vi "ELI-TriScope-StageController-V1.0.0.vi"() -> ()   [LabVIEW 2011]
uses:
  D:/Program Files/New Focus/New Focus Picomotor Application/Samples/CmdLib.dll
panel:
  in  "CurrentAngleA":dbl caption="CurrentAngle:" format="%.3g"
  in  "步长（nm）":dbl=31.75 format="%.2f"
  in  "relative position":i32=100
  in  "position profile":T1={"profileVelocity"=1000, "profileAcceleration"=10000, "profileDeceleration"=10000}
  in  "homeA":bool
  in  "ZeroA":bool
  in  "GoA":bool
  in  "AngleA":dbl=-18.0 caption="Angle:" format="%.3g"
  in  "file (use dialog)":path=path "C:/Users/Administrator/Desktop/stage2.txt"
  out "Current PositionY":dbl caption="Position:" format="%.3g"
  in  "JogY+":bool
  in  "JogY-":bool
  in  "StopY":bool
  in  "GoY":bool
  in  "Relative MoveY":dbl=3.0 caption="Step:" format="%.3g"
  out "Current PositionX":dbl caption="Position:" format="%.3g"
  in  "JogX+":bool
  in  "JogX-":bool
  in  "StopX":bool
  in  "GoX":bool
  in  "Relative MoveX":dbl=3.0 caption="Step:" format="%.3g"
  out "XYZ motors connect":bool
  in  "GoX 2":bool
  in  "GoY 2":bool
  in  "homeX":bool
  in  "ZeroX":bool
  in  "homeY":bool
  in  "ZeroY":bool
  out "Position:":dbl format="%.3g"
  in  "JogZ+":bool
  in  "JogZ-":bool
  in  "StopZ":bool
  in  "GoZ":bool
  in  "Relative MoveZ":dbl=3.0 caption="Step:" format="%.3g"
  in  "GoZ 2":bool
  in  "homeZ":bool
  in  "ZeroZ":bool
  out "targetPosZ":i32=88
  out "targetPosY":i32=13
  out "targetPosX":i32=-3455
  out "offsetZ":i32=-88
  out "offsetY":i32=-13
  out "offsetX":i32=3455
  out "CC Min":u32
  out "Exp. out":i32
  out "Clearing modes":i32=3
  out "Full CCD Height":i32=1200
  out "Full CCD Width":i32=1200
  out "Y Binning":u32=1
  out "X Binning":u32=1
  # "X motor"
  # "（um）"
  # "（um）"
  # "Y motor"
  # "（um）"
  # "（um）"
  # "Z motor"
  # "（um）"
  # "（um）"
  # "A motor"
  # "（°）"
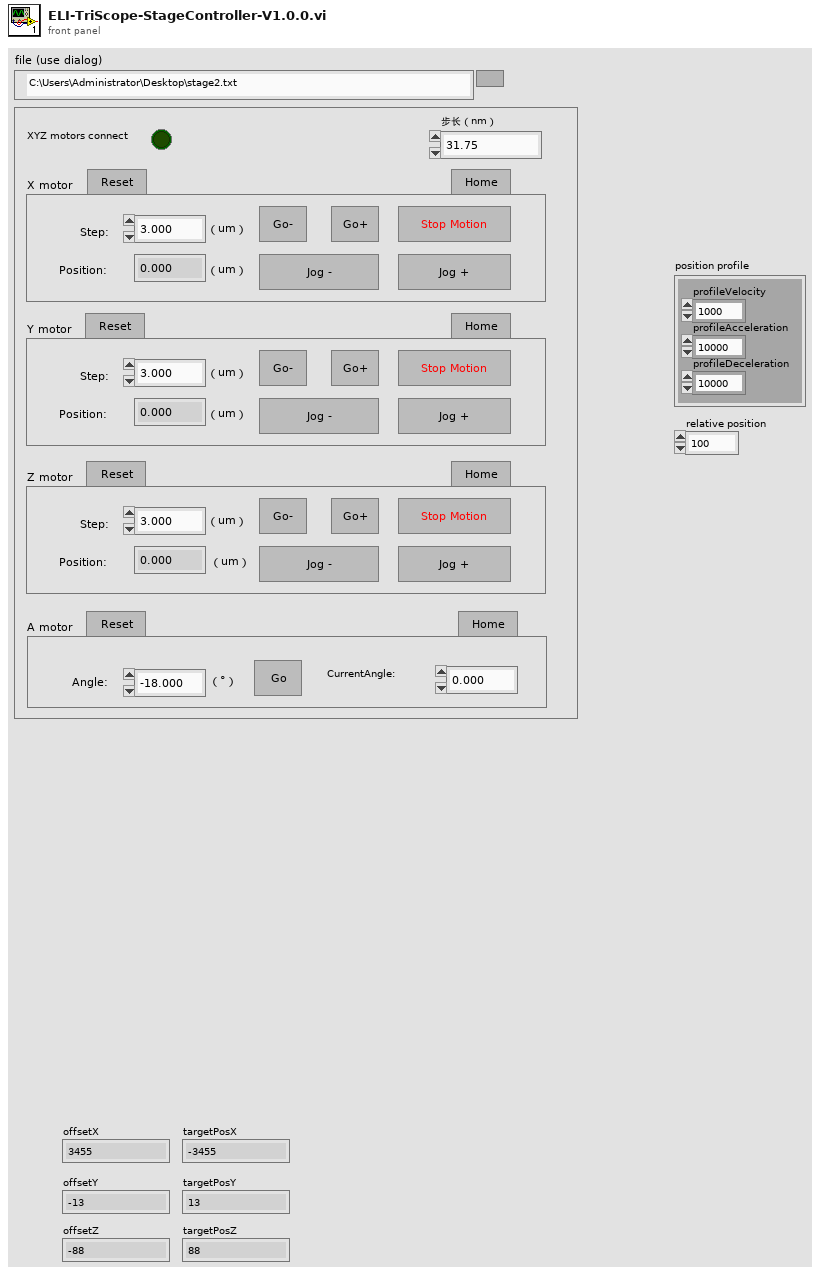
[diagram p1: front panel]
types:
  T1 = cluster{"profileVelocity":u32, "profileAcceleration":u32, "profileDeceleration":u32}
  T2 = cluster{"deviceName":string, "protocolStackName":string, "interfaceName":string, "portName":string, "baudrate":u32, "timeout":u32}
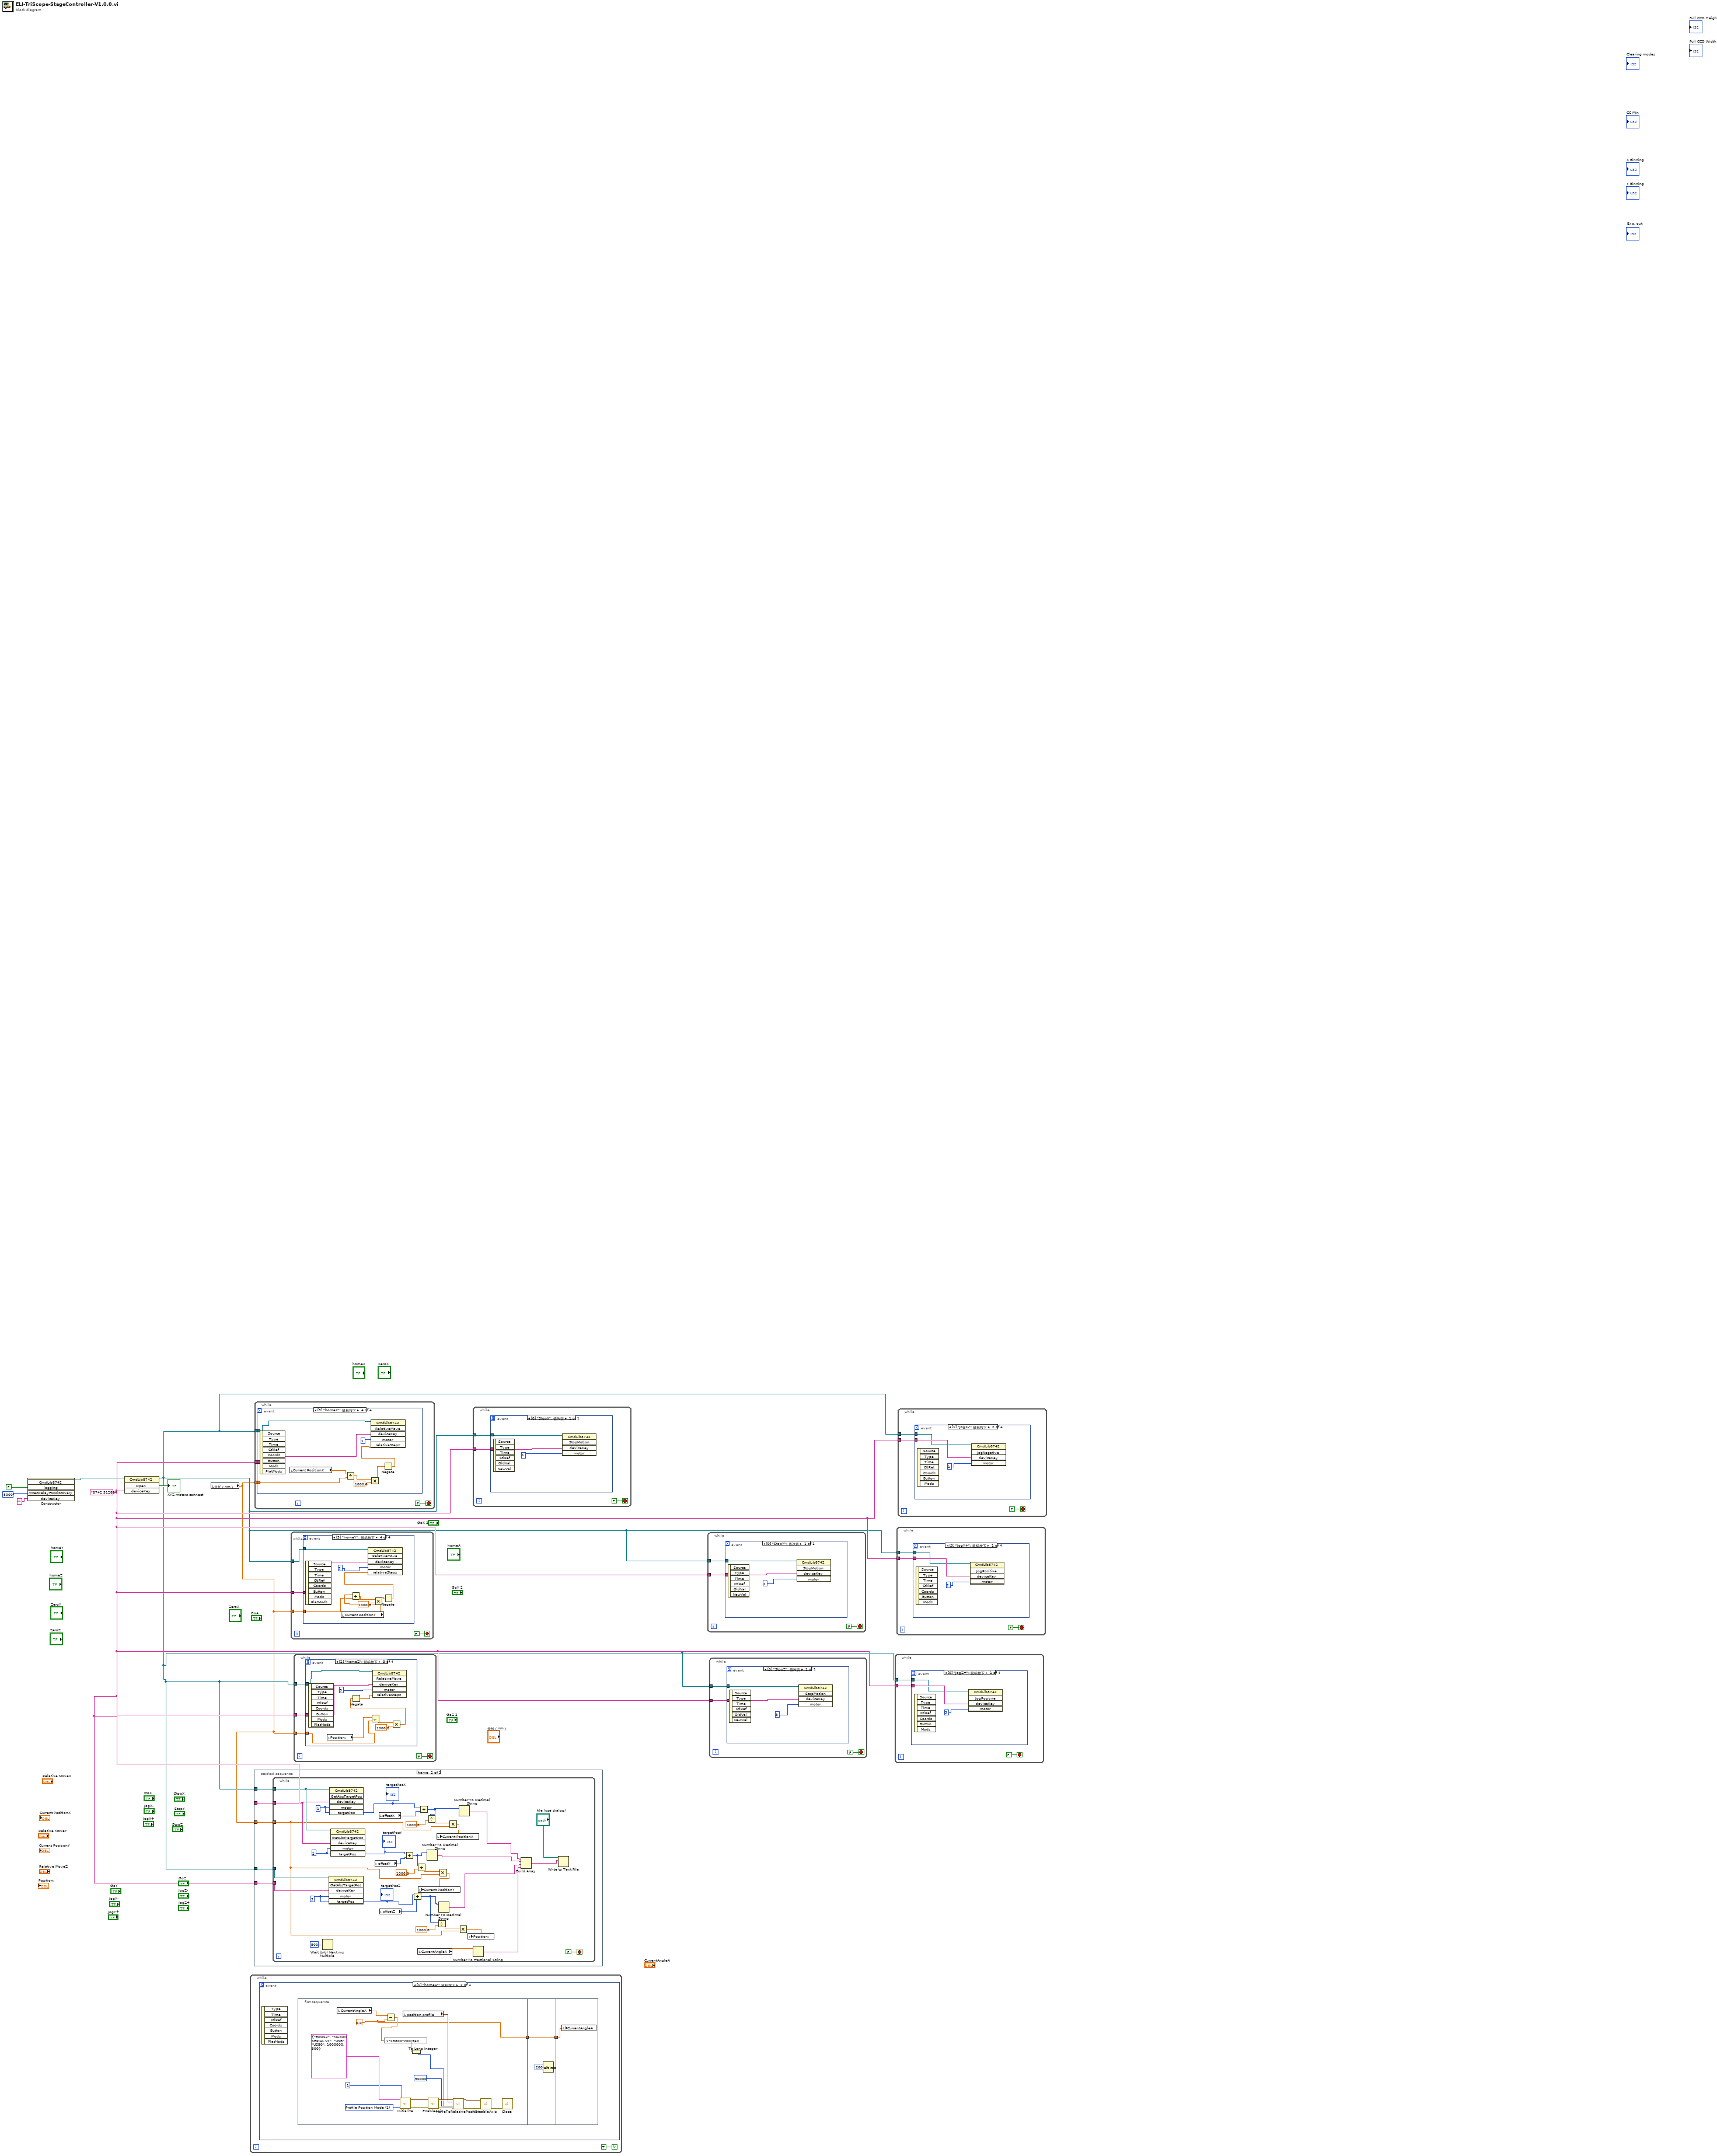
[diagram p0: block diagram]
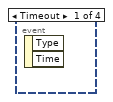
[diagram p2: hidden frame]
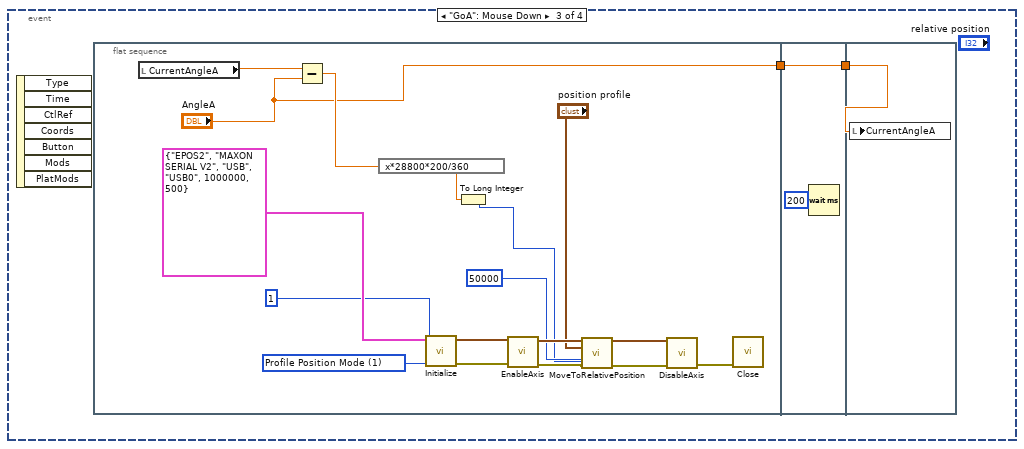
[diagram p3: hidden frame]
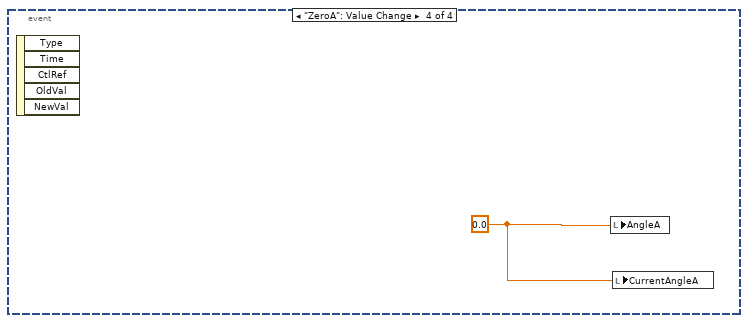
[diagram p4: hidden frame]
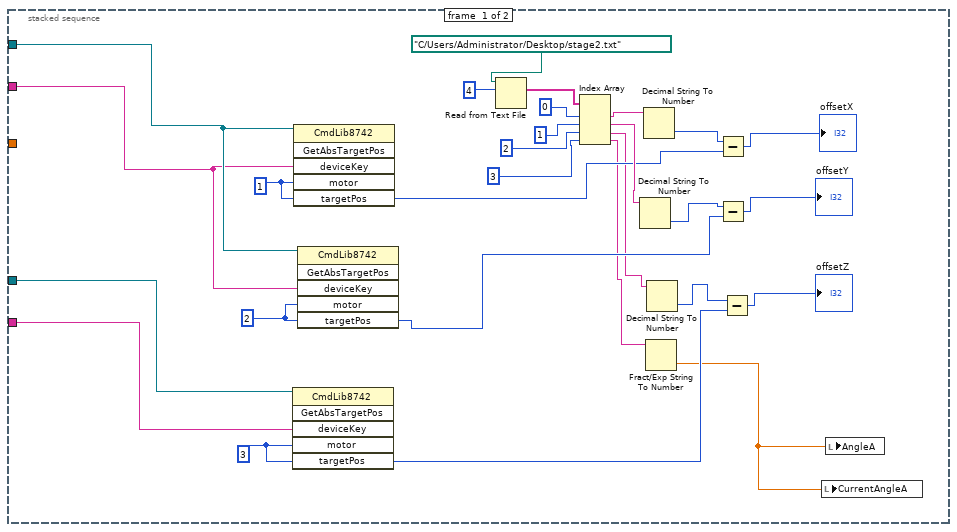
[diagram p5: hidden frame]
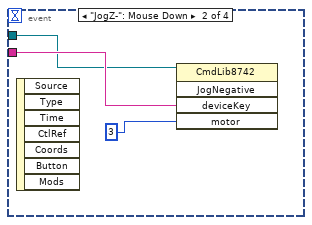
[diagram p6: hidden frame]
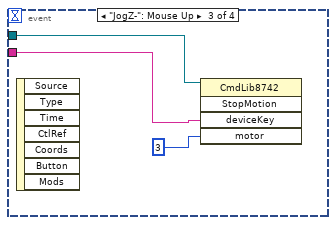
[diagram p7: hidden frame]
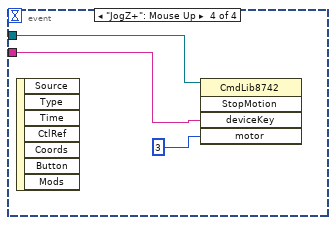
[diagram p8: hidden frame]
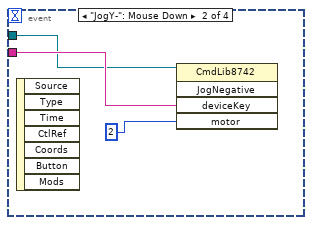
[diagram p9: hidden frame]
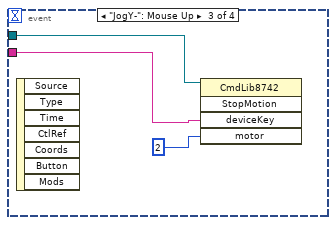
[diagram p10: hidden frame]
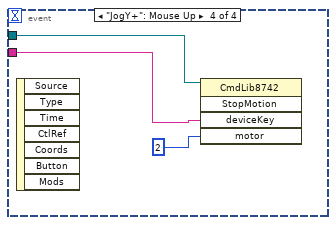
[diagram p11: hidden frame]
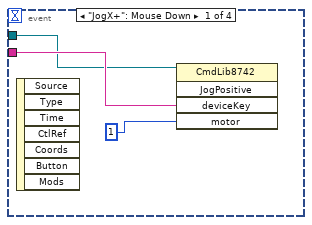
[diagram p12: hidden frame]
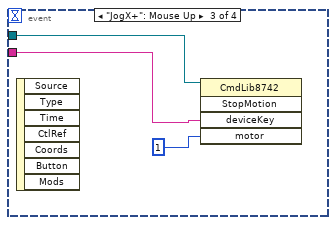
[diagram p13: hidden frame]
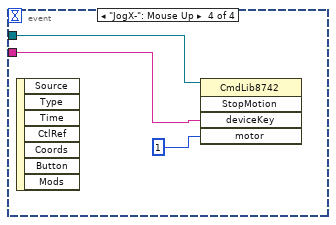
[diagram p14: hidden frame]
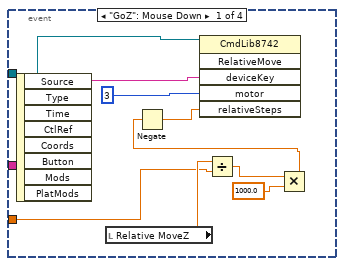
[diagram p15: hidden frame]
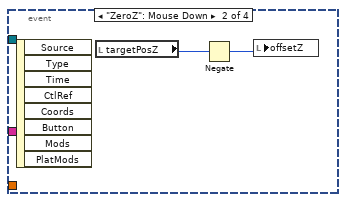
[diagram p16: hidden frame]
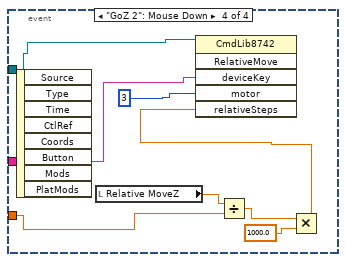
[diagram p17: hidden frame]
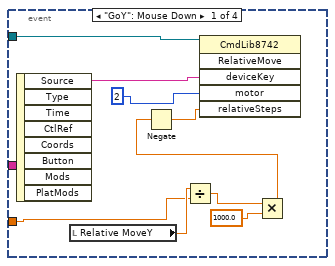
[diagram p18: hidden frame]
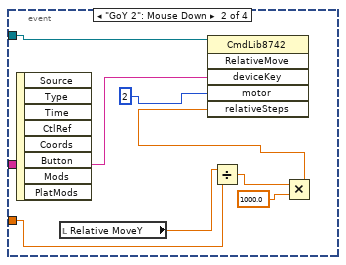
[diagram p19: hidden frame]
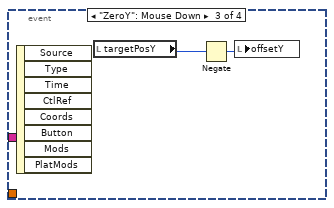
[diagram p20: hidden frame]
diagram:
  w3 = "8742 51285"
  n1 = constructor class="CmdLib8742"("logging"=FALSE, "msecDelayForDiscovery"=5000, "deviceKey"="") -> (reference out=w4:refnum<k24>)  [unwired: 3 in, 5 out]
  n2 = invoke class="CmdLib8742" method="Open"(reference=w4, "deviceKey"=w3) -> (reference out=w2:refnum<k24>, "Open"=→"XYZ motors connect":bool)  [unwired: 2 in, 2 out]
  n3 = local read "步长（nm）"() -> (w1:dbl)
  n4 = while {
    stop <- TRUE continue-if-true
    n5 = event shown="[1] \"homeA\": 鼠标按下" {
      selector: _ -> [_ _ _ _]
      dyn-events: _ -> [_ _ _ _]
      timeout: _ -> [_ _ _ _]
      event Timeout {
        n6 = event-data() -> ()  [unwired: 1 in, 2 out]
      }
      event "homeA": Mouse Down {
        n7 = event-data() -> ()  [unwired: 1 in, 7 out]
        n8 = flat-sequence {
          tunnel: [w12] -> w10
          tunnel: [w30] -> w11
          tunnel: w10 -> [w30]
          tunnel: w11 -> [w31]
          frame #0 {
            w12 = 0.0
            w27 = i8 1 items=["Profile Position Mode"=1, "Profile Velocity Mode"=3, "Homing Mode"=6, "Interpolated Position Mode"=7, "Position Mode"=-1, "Velocity Mode"=-2, "Current Mode"=-3, "Master Encoder Mode"=-5, "Step Direction Mode"=-6] ("modes of operations")
            n9 = local read "CurrentAngleA"() -> (w14:dbl)
            n10 = Subtract(x=w14, y=w12) -> (x-y=w13:dbl)
            n11 = expression code="x*28800*200/360"(w13) -> (w19:dbl)
            n12 = call "Initialize.vi"("modes of operations"=w27, "nodeId"=u16 1, "communication settings in"=T2 {"deviceName"="EPOS2", "protocolStackName"="MAXON SERIAL V2", "interfaceName"="USB", "portName"="USB0", "baudrate"=1000000, "timeout"=500}) -> ("error out"=w25:errorcluster, "axis out"=w22:cluster{"keyHandle":u32, "nodeId":u16})  [unwired: 7 in]
            n13 = local read "position profile"() -> (w17:T1)
            n14 = To Long Integer(number=w19) -> (32bit integer=w18:i32)
            n15 = call "EnableAxis.vi"("error in (no error)"=w25, "axis in"=w22) -> ("error out"=w24:errorcluster, "axis out"=w21:cluster{"keyHandle":u32, "nodeId":u16})  [unwired: 4 in]
            n16 = call "MoveToRelativePosition.vi"("axis in"=w21, "position profile"=w17, "relative position"=w18, "timeout"=u32 50000, "error in (no error)"=w24) -> ("axis out"=w16:cluster{"keyHandle":u32, "nodeId":u16}, "error out"=w23:errorcluster)  [unwired: 9 in]
            n17 = call "DisableAxis.vi"("error in (no error)"=w23, "axis in"=w16) -> ("error out"=w15:errorcluster)  [unwired: 4 in, 1 out]
            n18 = call "Close.vi"("error in (no error)"=w15) -> ()  [unwired: 10 in, 1 out]
          }
          frame #1 {
            n19 = Wait (ms)(milliseconds to wait=u32 200 ("等待时间（毫秒）")) -> ()  [unwired: 1 out]
          }
          frame #2 {
            n20 = local write "CurrentAngleA"(w31) -> ()
          }
        }
      }
      event "GoA": Mouse Down {
        n21 = event-data() -> ()  [unwired: 1 in, 7 out]
        n22 = flat-sequence {
          tunnel: ["AngleA"] -> w32
          tunnel: [w52] -> w33
          tunnel: w32 -> [w52]
          tunnel: w33 -> [w53]
          frame #0 {
            w49 = i8 1 items=["Profile Position Mode"=1, "Profile Velocity Mode"=3, "Homing Mode"=6, "Interpolated Position Mode"=7, "Position Mode"=-1, "Velocity Mode"=-2, "Current Mode"=-3, "Master Encoder Mode"=-5, "Step Direction Mode"=-6] ("modes of operations")
            n23 = local read "CurrentAngleA"() -> (w36:dbl)
            n24 = Subtract(x=w36, y="AngleA") -> (x-y=w35:dbl)
            n25 = expression code="x*28800*200/360"(w35) -> (w41:dbl)
            n26 = call "Initialize.vi"("modes of operations"=w49, "nodeId"=u16 1, "communication settings in"=T2 {"deviceName"="EPOS2", "protocolStackName"="MAXON SERIAL V2", "interfaceName"="USB", "portName"="USB0", "baudrate"=1000000, "timeout"=500}) -> ("error out"=w47:errorcluster, "axis out"=w45:cluster{"keyHandle":u32, "nodeId":u16})  [unwired: 7 in]
            n27 = To Long Integer(number=w41) -> (32bit integer=w40:i32)
            n28 = call "EnableAxis.vi"("error in (no error)"=w47, "axis in"=w45) -> ("error out"=w46:errorcluster, "axis out"=w44:cluster{"keyHandle":u32, "nodeId":u16})  [unwired: 4 in]
            n29 = call "MoveToRelativePosition.vi"("axis in"=w44, "position profile"="position profile", "relative position"=w40, "timeout"=u32 50000, "error in (no error)"=w46) -> ("axis out"=w39:cluster{"keyHandle":u32, "nodeId":u16}, "error out"=w38:errorcluster)  [unwired: 9 in]
            n30 = call "DisableAxis.vi"("error in (no error)"=w38, "axis in"=w39) -> ("error out"=w37:errorcluster)  [unwired: 4 in, 1 out]
            n31 = call "Close.vi"("error in (no error)"=w37) -> ()  [unwired: 10 in, 1 out]
          }
          frame #1 {
            n32 = Wait (ms)(milliseconds to wait=u32 200 ("等待时间（毫秒）")) -> ()  [unwired: 1 out]
          }
          frame #2 {
            n33 = local write "CurrentAngleA"(w53) -> ()
          }
        }
      }
      event "ZeroA": Value Change {
        w54 = 0.0 ("AngleA")
        n34 = event-data() -> ()  [unwired: 1 in, 5 out]
        n35 = local write "AngleA"(w54) -> ()
        n36 = local write "CurrentAngleA"(w54) -> ()
      }
    }
  }
  n37 = stacked-sequence {
    tunnel: w2 -> [w72 w87]
    tunnel: w3 -> [w71 w86]
    tunnel: w2 -> [w70 w85]
    tunnel: w3 -> [w69 w84]
    tunnel: w1 -> [_ w83]
    frame #0 {
      w73 = 2 ("motor")
      w74 = 1 ("motor")
      w75 = 3 ("motor")
      n38 = invoke class="CmdLib8742" method="GetAbsTargetPos"(reference=w70, "deviceKey"=w69, "motor"=w75, "targetPos"=w75) -> ("targetPos"=w61:i32)  [unwired: 2 in, 5 out]
      n39 = invoke class="CmdLib8742" method="GetAbsTargetPos"(reference=w72, "deviceKey"=w71, "motor"=w74, "targetPos"=w74) -> ("targetPos"=w67:i32)  [unwired: 2 in, 5 out]
      n40 = invoke class="CmdLib8742" method="GetAbsTargetPos"(reference=w72, "deviceKey"=w71, "motor"=w73, "targetPos"=w73) -> ("targetPos"=w64:i32)  [unwired: 2 in, 5 out]
      n41 = Read from Text File(file (use dialog)=path "C:/Users/Administrator/Desktop/stage2.txt", count=4 ("index")) -> (text=w79:string[])  [unwired: 2 in, 3 out]
      n42 = Index Array(array=w79, index #1=0 ("index"), index #2=1 ("index"), index #3=2 ("index"), index #4=3 ("index")) -> (element #1=w82:string, element #2=w76:string, element #3=w57:string, element #4=w56:string)
      n43 = Decimal String To Number(string=w76) -> (number=w65:i32)  [unwired: 2 in, 1 out]
      n44 = Decimal String To Number(string=w82) -> (number=w68:i32)  [unwired: 2 in, 1 out]
      n45 = Fract/Exp String To Number(string=w56) -> (number=w55:dbl)  [unwired: 3 in, 1 out]
      n46 = Decimal String To Number(string=w57) -> (number=w62:i32)  [unwired: 2 in, 1 out]
      n47 = Subtract(x=w68, y=w67) -> (x-y=→"offsetX":i32)
      n48 = Subtract(x=w65, y=w64) -> (x-y=→"offsetY":i32)
      n49 = Subtract(x=w62, y=w61) -> (x-y=→"offsetZ":i32)
      n50 = local write "CurrentAngleA"(w55) -> ()
      n51 = local write "AngleA"(w55) -> ()
    }
    frame #1 {
      n52 = while {
        tunnel: w85 -> [w122]
        tunnel: w84 -> [w121]
        tunnel: w87 -> [w116]
        tunnel: w86 -> [w115]
        tunnel: w83 -> [w92]
        stop <- FALSE stop-if-true
        w114 = 2 ("motor")
        w117 = 1 ("motor")
        w118 = 3 ("motor")
        n53 = Wait Until Next ms Multiple(millisecond multiple=500) -> ()  [unwired: 1 out]
        n54 = invoke class="CmdLib8742" method="GetAbsTargetPos"(reference=w122, "deviceKey"=w121, "motor"=w118, "targetPos"=w118) -> ("targetPos"=w108:i32)  [unwired: 2 in, 5 out]
        "targetPosZ" <- w108
        n55 = invoke class="CmdLib8742" method="GetAbsTargetPos"(reference=w116, "deviceKey"=w115, "motor"=w117, "targetPos"=w117) -> ("targetPos"=w111:i32)  [unwired: 2 in, 5 out]
        "targetPosX" <- w111
        n56 = invoke class="CmdLib8742" method="GetAbsTargetPos"(reference=w116, "deviceKey"=w115, "motor"=w114, "targetPos"=w114) -> ("targetPos"=w109:i32)  [unwired: 2 in, 5 out]
        "targetPosY" <- w109
        n57 = local read "offsetY"() -> (w107:i32)
        n58 = local read "offsetX"() -> (w110:i32)
        n59 = local read "offsetZ"() -> (w104:i32)
        n60 = Add(x=w109, y=w107) -> (x+y=w94:i32)
        n61 = Add(x=w108, y=w104) -> (x+y=w91:i32)
        n62 = Divide(x=w94, y=1000.0) -> (x/y=w98:dbl)
        n63 = local read "CurrentAngleA"() -> (w88:dbl)
        n64 = Add(x=w111, y=w110) -> (x+y=w100:i32)
        n65 = Divide(x=w100, y=1000.0) -> (x/y=w102:dbl)
        n66 = Number To Decimal String(number=w94) -> (decimal integer string=w105:string)  [unwired: 1 in]
        n67 = Divide(x=w91, y=1000.0) -> (x/y=w96:dbl)
        n68 = Multiply(x=w98, y=w92) -> (x*y=w93:dbl)
        n69 = local write "Current PositionY"(w93) -> ()
        n70 = Number To Decimal String(number=w91) -> (decimal integer string=w103:string)  [unwired: 1 in]
        n71 = Multiply(x=w102, y=w92) -> (x*y=w99:dbl)
        n72 = local write "Current PositionX"(w99) -> ()
        n73 = Multiply(x=w96, y=w92) -> (x*y=w90:dbl)
        n74 = Number To Decimal String(number=w100) -> (decimal integer string=w106:string)  [unwired: 1 in]
        n75 = local write "Position:"(w90) -> ()
        n76 = Number To Fractional String(number=w88) -> (F-format string=w89:string)  [unwired: 3 in]
        n77 = Build Array(w106, w105, w103, w89) -> (w113:string[])
        n78 = Write to Text File(file (use dialog)="file (use dialog)", text=w113) -> ()  [unwired: 2 in, 3 out]
      }
    }
  }
  n79 = while {
    tunnel: w2 -> [w126]
    tunnel: w3 -> [w125]
    tunnel: w1 -> [w123]
    stop <- FALSE stop-if-true
    n80 = event shown="[3] \"homeX\": 鼠标按下" {
      selector: _ -> [_ _ _ _]
      dyn-events: _ -> [_ _ _ _]
      timeout: _ -> [_ _ _ _]
      tunnel: w126 -> [w135 w143 _ w152]
      tunnel: w125 -> [w134 w141 _ w153]
      tunnel: w123 -> [w127 w137 _ w146]
      event "GoX": Mouse Down {
        n81 = event-data() -> ()  [unwired: 1 in, 8 out]
        n82 = local read "Relative MoveX"() -> (w129:dbl)
        n83 = Divide(x=w129, y=w127) -> (x/y=w131:dbl)
        n84 = Multiply(x=w131, y=1000.0) -> (x*y=w128:dbl)
        n85 = Negate(x=w128) -> (-x=w132:dbl)
        n86 = invoke class="CmdLib8742" method="RelativeMove"(reference=w135, "deviceKey"=w134, "motor"=1, "relativeSteps"=w132) -> ()  [unwired: 2 in, 6 out]
      }
      event "GoX 2": Mouse Down {
        n87 = event-data() -> ()  [unwired: 1 in, 8 out]
        n88 = local read "Relative MoveX"() -> (w138:dbl)
        n89 = Divide(x=w138, y=w137) -> (x/y=w140:dbl)
        n90 = Multiply(x=w140, y=1000.0) -> (x*y=w136:dbl)
        n91 = invoke class="CmdLib8742" method="RelativeMove"(reference=w143, "deviceKey"=w141, "motor"=1, "relativeSteps"=w136) -> ()  [unwired: 2 in, 6 out]
      }
      event "ZeroX": Mouse Down {
        n92 = event-data() -> ()  [unwired: 1 in, 8 out]
        n93 = local read "targetPosX"() -> (w145:i32)
        n94 = Negate(x=w145) -> (-x=w144:i32)
        n95 = local write "offsetX"(w144) -> ()
      }
      event "homeX": Mouse Down {
        n96 = event-data() -> ()  [unwired: 1 in, 8 out]
        n97 = local read "Current PositionX"() -> (w150:dbl)
        n98 = Divide(x=w150, y=w146) -> (x/y=w149:dbl)
        n99 = Multiply(x=w149, y=1000.0) -> (x*y=w147:dbl)
        n100 = Negate(x=w147) -> (-x=w151:dbl)
        n101 = invoke class="CmdLib8742" method="RelativeMove"(reference=w152, "deviceKey"=w153, "motor"=1, "relativeSteps"=w151) -> ()  [unwired: 2 in, 6 out]
      }
    }
  }
  n102 = while {
    tunnel: w2 -> [w158]
    tunnel: w3 -> [w157]
    tunnel: w1 -> [w155]
    stop <- FALSE stop-if-true
    n103 = event shown="[3] \"homeY\": 鼠标按下" {
      selector: _ -> [_ _ _ _]
      dyn-events: _ -> [_ _ _ _]
      timeout: _ -> [_ _ _ _]
      tunnel: w158 -> [w167 w174 _ w185]
      tunnel: w157 -> [w166 w173 _ w184]
      tunnel: w155 -> [w160 w169 _ w178]
      event "GoY": Mouse Down {
        n104 = event-data() -> ()  [unwired: 1 in, 8 out]
        n105 = local read "Relative MoveY"() -> (w161:dbl)
        n106 = Divide(x=w161, y=w160) -> (x/y=w163:dbl)
        n107 = Multiply(x=w163, y=1000.0) -> (x*y=w159:dbl)
        n108 = Negate(x=w159) -> (-x=w164:dbl)
        n109 = invoke class="CmdLib8742" method="RelativeMove"(reference=w167, "deviceKey"=w166, "motor"=2, "relativeSteps"=w164) -> ()  [unwired: 2 in, 6 out]
      }
      event "GoY 2": Mouse Down {
        n110 = event-data() -> ()  [unwired: 1 in, 8 out]
        n111 = local read "Relative MoveY"() -> (w170:dbl)
        n112 = Divide(x=w170, y=w169) -> (x/y=w172:dbl)
        n113 = Multiply(x=w172, y=1000.0) -> (x*y=w168:dbl)
        n114 = invoke class="CmdLib8742" method="RelativeMove"(reference=w174, "deviceKey"=w173, "motor"=2, "relativeSteps"=w168) -> ()  [unwired: 2 in, 6 out]
      }
      event "ZeroY": Mouse Down {
        n115 = event-data() -> ()  [unwired: 1 in, 8 out]
        n116 = local read "targetPosY"() -> (w176:i32)
        n117 = Negate(x=w176) -> (-x=w177:i32)
        n118 = local write "offsetY"(w177) -> ()
      }
      event "homeY": Mouse Down {
        n119 = event-data() -> ()  [unwired: 1 in, 8 out]
        n120 = local read "Current PositionY"() -> (w180:dbl)
        n121 = Divide(x=w180, y=w178) -> (x/y=w182:dbl)
        n122 = Multiply(x=w182, y=1000.0) -> (x*y=w179:dbl)
        n123 = Negate(x=w179) -> (-x=w183:dbl)
        n124 = invoke class="CmdLib8742" method="RelativeMove"(reference=w185, "deviceKey"=w184, "motor"=2, "relativeSteps"=w183) -> ()  [unwired: 2 in, 6 out]
      }
    }
  }
  n125 = while {
    tunnel: w2 -> [w190]
    tunnel: w3 -> [w189]
    tunnel: w1 -> [w187]
    stop <- FALSE stop-if-true
    n126 = event shown="[2] \"homeZ\": 鼠标按下" {
      selector: _ -> [_ _ _ _]
      dyn-events: _ -> [_ _ _ _]
      timeout: _ -> [_ _ _ _]
      tunnel: w190 -> [w199 _ w208 w217]
      tunnel: w189 -> [w198 _ w207 w216]
      tunnel: w187 -> [w192 _ w202 w212]
      event "GoZ": Mouse Down {
        n127 = event-data() -> ()  [unwired: 1 in, 8 out]
        n128 = local read "Relative MoveZ"() -> (w193:dbl)
        n129 = Divide(x=w193, y=w192) -> (x/y=w195:dbl)
        n130 = Multiply(x=w195, y=1000.0) -> (x*y=w191:dbl)
        n131 = Negate(x=w191) -> (-x=w196:dbl)
        n132 = invoke class="CmdLib8742" method="RelativeMove"(reference=w199, "deviceKey"=w198, "motor"=3, "relativeSteps"=w196) -> ()  [unwired: 2 in, 6 out]
      }
      event "ZeroZ": Mouse Down {
        n133 = event-data() -> ()  [unwired: 1 in, 8 out]
        n134 = local read "targetPosZ"() -> (w200:i32)
        n135 = Negate(x=w200) -> (-x=w201:i32)
        n136 = local write "offsetZ"(w201) -> ()
      }
      event "homeZ": Mouse Down {
        n137 = event-data() -> ()  [unwired: 1 in, 8 out]
        n138 = local read "Position:"() -> (w204:dbl)
        n139 = Divide(x=w204, y=w202) -> (x/y=w206:dbl)
        n140 = Multiply(x=w206, y=1000.0) -> (x*y=w203:dbl)
        n141 = Negate(x=w203) -> (-x=w209:dbl)
        n142 = invoke class="CmdLib8742" method="RelativeMove"(reference=w208, "deviceKey"=w207, "motor"=3, "relativeSteps"=w209) -> ()  [unwired: 2 in, 6 out]
      }
      event "GoZ 2": Mouse Down {
        n143 = event-data() -> ()  [unwired: 1 in, 8 out]
        n144 = local read "Relative MoveZ"() -> (w213:dbl)
        n145 = Divide(x=w213, y=w212) -> (x/y=w215:dbl)
        n146 = Multiply(x=w215, y=1000.0) -> (x*y=w211:dbl)
        n147 = invoke class="CmdLib8742" method="RelativeMove"(reference=w217, "deviceKey"=w216, "motor"=3, "relativeSteps"=w211) -> ()  [unwired: 2 in, 6 out]
      }
    }
  }
  n148 = while {
    tunnel: w2 -> [w221]
    tunnel: w3 -> [w220]
    stop <- FALSE stop-if-true
    n149 = event shown="[0] \"StopX\": 值改变" {
      selector: _ -> [_]
      dyn-events: _ -> [_]
      timeout: _ -> [_]
      tunnel: w221 -> [w224]
      tunnel: w220 -> [w223]
      event "StopX": Value Change {
        n150 = event-data() -> ()  [unwired: 1 in, 6 out]
        n151 = invoke class="CmdLib8742" method="StopMotion"(reference=w224, "deviceKey"=w223, "motor"=1) -> ()  [unwired: 2 in, 5 out]
      }
    }
  }
  n152 = while {
    tunnel: w2 -> [w227]
    tunnel: w3 -> [w226]
    stop <- FALSE stop-if-true
    n153 = event shown="[0] \"StopY\": 值改变" {
      selector: _ -> [_]
      dyn-events: _ -> [_]
      timeout: _ -> [_]
      tunnel: w227 -> [w230]
      tunnel: w226 -> [w229]
      event "StopY": Value Change {
        n154 = event-data() -> ()  [unwired: 1 in, 6 out]
        n155 = invoke class="CmdLib8742" method="StopMotion"(reference=w230, "deviceKey"=w229, "motor"=2) -> ()  [unwired: 2 in, 5 out]
      }
    }
  }
  n156 = while {
    tunnel: w2 -> [w233]
    tunnel: w3 -> [w232]
    stop <- FALSE stop-if-true
    n157 = event shown="[0] \"StopZ\": 值改变" {
      selector: _ -> [_]
      dyn-events: _ -> [_]
      timeout: _ -> [_]
      tunnel: w233 -> [w236]
      tunnel: w232 -> [w235]
      event "StopZ": Value Change {
        n158 = event-data() -> ()  [unwired: 1 in, 6 out]
        n159 = invoke class="CmdLib8742" method="StopMotion"(reference=w236, "deviceKey"=w235, "motor"=3) -> ()  [unwired: 2 in, 5 out]
      }
    }
  }
  n160 = while {
    tunnel: w3 -> [w239]
    tunnel: w2 -> [w238]
    stop <- FALSE stop-if-true
    n161 = event shown="[0] \"JogZ+\": 鼠标按下" {
      selector: _ -> [_ _ _ _]
      dyn-events: _ -> [_ _ _ _]
      timeout: _ -> [_ _ _ _]
      tunnel: w239 -> [w242 w245 w247 w250]
      tunnel: w238 -> [w241 w244 w248 w251]
      event "JogZ+": Mouse Down {
        n162 = event-data() -> ()  [unwired: 1 in, 7 out]
        n163 = invoke class="CmdLib8742" method="JogPositive"(reference=w241, "deviceKey"=w242, "motor"=3) -> ()  [unwired: 2 in, 5 out]
      }
      event "JogZ-": Mouse Down {
        n164 = event-data() -> ()  [unwired: 1 in, 7 out]
        n165 = invoke class="CmdLib8742" method="JogNegative"(reference=w244, "deviceKey"=w245, "motor"=3) -> ()  [unwired: 2 in, 5 out]
      }
      event "JogZ-": Mouse Up {
        n166 = event-data() -> ()  [unwired: 1 in, 7 out]
        n167 = invoke class="CmdLib8742" method="StopMotion"(reference=w248, "deviceKey"=w247, "motor"=3) -> ()  [unwired: 2 in, 5 out]
      }
      event "JogZ+": Mouse Up {
        n168 = event-data() -> ()  [unwired: 1 in, 7 out]
        n169 = invoke class="CmdLib8742" method="StopMotion"(reference=w251, "deviceKey"=w250, "motor"=3) -> ()  [unwired: 2 in, 5 out]
      }
    }
  }
  n170 = while {
    tunnel: w3 -> [w254]
    tunnel: w2 -> [w253]
    stop <- FALSE stop-if-true
    n171 = event shown="[0] \"JogY+\": 鼠标按下" {
      selector: _ -> [_ _ _ _]
      dyn-events: _ -> [_ _ _ _]
      timeout: _ -> [_ _ _ _]
      tunnel: w254 -> [w257 w260 w262 w265]
      tunnel: w253 -> [w256 w259 w263 w266]
      event "JogY+": Mouse Down {
        n172 = event-data() -> ()  [unwired: 1 in, 7 out]
        n173 = invoke class="CmdLib8742" method="JogPositive"(reference=w256, "deviceKey"=w257, "motor"=2) -> ()  [unwired: 2 in, 5 out]
      }
      event "JogY-": Mouse Down {
        n174 = event-data() -> ()  [unwired: 1 in, 7 out]
        n175 = invoke class="CmdLib8742" method="JogNegative"(reference=w259, "deviceKey"=w260, "motor"=2) -> ()  [unwired: 2 in, 5 out]
      }
      event "JogY-": Mouse Up {
        n176 = event-data() -> ()  [unwired: 1 in, 7 out]
        n177 = invoke class="CmdLib8742" method="StopMotion"(reference=w263, "deviceKey"=w262, "motor"=2) -> ()  [unwired: 2 in, 5 out]
      }
      event "JogY+": Mouse Up {
        n178 = event-data() -> ()  [unwired: 1 in, 7 out]
        n179 = invoke class="CmdLib8742" method="StopMotion"(reference=w266, "deviceKey"=w265, "motor"=2) -> ()  [unwired: 2 in, 5 out]
      }
    }
  }
  n180 = while {
    tunnel: w3 -> [w269]
    tunnel: w2 -> [w268]
    stop <- FALSE stop-if-true
    n181 = event shown="[1] \"JogX-\": 鼠标按下" {
      selector: _ -> [_ _ _ _]
      dyn-events: _ -> [_ _ _ _]
      timeout: _ -> [_ _ _ _]
      tunnel: w269 -> [w272 w275 w277 w280]
      tunnel: w268 -> [w271 w274 w278 w281]
      event "JogX+": Mouse Down {
        n182 = event-data() -> ()  [unwired: 1 in, 7 out]
        n183 = invoke class="CmdLib8742" method="JogPositive"(reference=w271, "deviceKey"=w272, "motor"=1) -> ()  [unwired: 2 in, 5 out]
      }
      event "JogX-": Mouse Down {
        n184 = event-data() -> ()  [unwired: 1 in, 7 out]
        n185 = invoke class="CmdLib8742" method="JogNegative"(reference=w274, "deviceKey"=w275, "motor"=1) -> ()  [unwired: 2 in, 5 out]
      }
      event "JogX+": Mouse Up {
        n186 = event-data() -> ()  [unwired: 1 in, 7 out]
        n187 = invoke class="CmdLib8742" method="StopMotion"(reference=w278, "deviceKey"=w277, "motor"=1) -> ()  [unwired: 2 in, 5 out]
      }
      event "JogX-": Mouse Up {
        n188 = event-data() -> ()  [unwired: 1 in, 7 out]
        n189 = invoke class="CmdLib8742" method="StopMotion"(reference=w281, "deviceKey"=w280, "motor"=1) -> ()  [unwired: 2 in, 5 out]
      }
    }
  }
